vi "test5.vi"() -> ()   [LabVIEW 2014]
panel:
  out "In Range?":bool
  out "x-y":u32
  out "millisecond timer value 2":u32
  out "element":u32
  out "s? t:f 3":string
  out "s? t:f 2":string
  out "s? t:f":string
  out "appended array":u32[](array[numeric])
  out "millisecond timer value":u32
  in  "stop 2":bool
  out "String":string="3"
  out "Boolean 3":bool
  out "Boolean 2":bool
  out "Boolean":bool
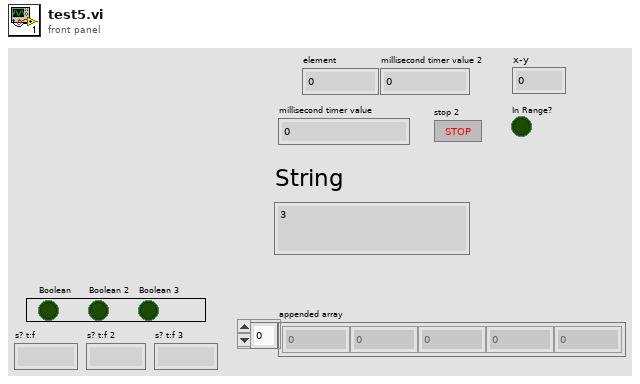
[diagram p1: front panel]
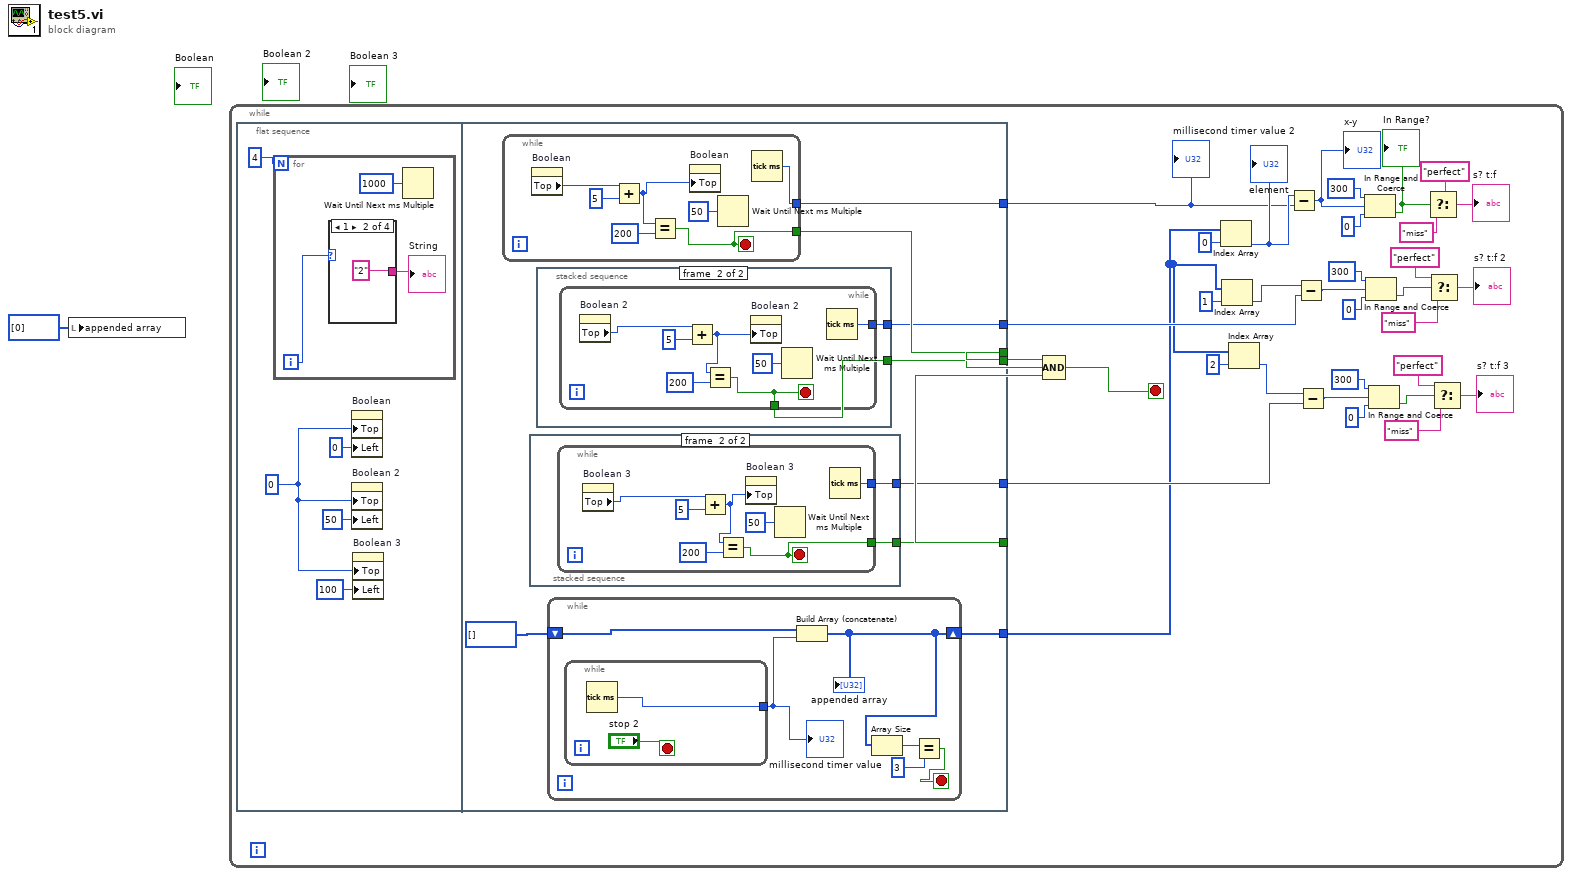
[diagram p0: block diagram]
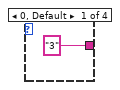
[diagram p2: hidden frame]
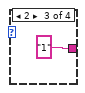
[diagram p3: hidden frame]
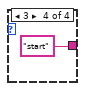
[diagram p4: hidden frame]
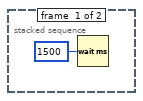
[diagram p5: hidden frame]
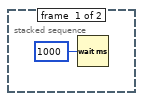
[diagram p6: hidden frame]
diagram:
  n1 = local write "appended array"(u32[] [0] ("appended array")) -> ()
  n2 = while {
    stop <- w33 stop-if-true
    n3 = flat-sequence {
      tunnel: [w56] -> w36
      tunnel: [w55] -> w35
      tunnel: [w54] -> w34
      tunnel: [w53] -> w28
      tunnel: [w52] -> w27
      tunnel: [w51] -> w25
      tunnel: [w49] -> w2
      frame #0 {
        w39 = 0
        n4 = for {
          N: 4 -> [_]
          i -> [w44]
          n5 = case shown="1" w44 {
            tunnel: ["3" "2" "1" "start"] -> w42
            frame 0, Default {
            }
            frame 1 {
            }
            frame 2 {
            }
            frame 3 {
            }
          }
          "String" <- w42
          n6 = Wait Until Next ms Multiple(millisecond multiple=u32 1000) -> ()  [unwired: 1 out]
        }
        n7 = property on="Boolean" class="Bool (strict)"("Top"=w39, "Left"=0 ("Position:Left")) -> ()  [unwired: 2 in, 2 out]
        n8 = property on="Boolean 2" class="Bool (strict)"("Top"=w39, "Left"=50 ("Position:Left")) -> ()  [unwired: 2 in, 2 out]
        n9 = property on="Boolean 3" class="Bool (strict)"("Top"=w39, "Left"=100 ("Position:Left")) -> ()  [unwired: 2 in, 2 out]
      }
      frame #1 {
        n10 = while {
          tunnel: [w86] -> w56
          tunnel: [w85] -> w53
          stop <- w86 stop-if-true
          n11 = property on="Boolean" class="Bool (strict)"() -> ("Top"=w90:i32)  [unwired: 2 in, 2 out]
          n12 = Add(x=w90, y=5) -> (x+y=w88:i32)
          n13 = Equal?(x=w88, y=200) -> (x = y?=w86:bool)
          n14 = property on="Boolean" class="Bool (strict)"("Top"=w88) -> ()  [unwired: 2 in, 2 out]
          n15 = Wait Until Next ms Multiple(millisecond multiple=u32 50) -> ()  [unwired: 1 out]
          n16 = Tick Count (ms)() -> (millisecond timer value=w85:u32)
        }
        n17 = stacked-sequence {
          tunnel: [_ w67] -> w54
          tunnel: [_ w66] -> w51
          frame #0 {
            n18 = Wait (ms)(milliseconds to wait=u32 1500) -> ()  [unwired: 1 out]
          }
          frame #1 {
            n19 = while {
              tunnel: [w70] -> w67
              tunnel: [w68] -> w66
              stop <- w70 stop-if-true
              n20 = property on="Boolean 3" class="Bool (strict)"() -> ("Top"=w71:i32)  [unwired: 2 in, 2 out]
              n21 = Add(x=w71, y=5) -> (x+y=w69:i32)
              n22 = Equal?(x=w69, y=200) -> (x = y?=w70:bool)
              n23 = property on="Boolean 3" class="Bool (strict)"("Top"=w69) -> ()  [unwired: 2 in, 2 out]
              n24 = Wait Until Next ms Multiple(millisecond multiple=u32 50) -> ()  [unwired: 1 out]
              n25 = Tick Count (ms)() -> (millisecond timer value=w68:u32)
            }
          }
        }
        n26 = stacked-sequence {
          tunnel: [_ w77] -> w55
          tunnel: [_ w76] -> w52
          frame #0 {
            n27 = Wait (ms)(milliseconds to wait=u32 1000) -> ()  [unwired: 1 out]
          }
          frame #1 {
            n28 = while {
              tunnel: [w79] -> w77
              tunnel: [w78] -> w76
              stop <- w79 stop-if-true
              n29 = property on="Boolean 2" class="Bool (strict)"() -> ("Top"=w82:i32)  [unwired: 2 in, 2 out]
              n30 = Add(x=w82, y=5) -> (x+y=w80:i32)
              n31 = Equal?(x=w80, y=200) -> (x = y?=w79:bool)
              n32 = property on="Boolean 2" class="Bool (strict)"("Top"=w80) -> ()  [unwired: 2 in, 2 out]
              n33 = Wait Until Next ms Multiple(millisecond multiple=u32 50) -> ()  [unwired: 1 out]
              n34 = Tick Count (ms)() -> (millisecond timer value=w78:u32)
            }
          }
        }
        n35 = while {
          shift-right: [w60] -> w49
          shift-left: u32[] [] -> [w62]
          stop <- w57 stop-if-true
          n36 = while {
            tunnel: [w63] -> w61
            stop <- "stop 2" stop-if-true
            n37 = Tick Count (ms)() -> (millisecond timer value=w63:u32)
          }
          "millisecond timer value" <- w61
          n38 = Build Array (concatenate)(w62, w61) -> (w60:u32[])
          "appended array" <- w60
          n39 = Array Size(array=w60) -> (size(s)=w59:i32)
          n40 = Equal?(x=w59, y=3) -> (x = y?=w57:bool)
        }
      }
    }
    n41 = Compound Arithmetic op=AND(w36, w35, w34) -> (w33:bool)
    n42 = Index Array(array=w2, index=0) -> (element=w29:u32)
    "element" <- w29
    n43 = Index Array(array=w2, index=1) -> (element=w26:u32)
    n44 = Index Array(array=w2, index=2) -> (element=w24:u32)
    n45 = Subtract(x=w29, y=w28) -> (x-y=w23:u32)
    "x-y" <- w23
    n46 = Subtract(x=w26, y=w27) -> (x-y=w4:u32)
    n47 = Subtract(x=w24, y=w25) -> (x-y=w3:u32)
    n48 = In Range and Coerce(upper limit=u32 300, x=w23, lower limit=u32 0) -> (In Range?=w20:bool)  [unwired: 1 out]
    "In Range?" <- w20
    n49 = In Range and Coerce(upper limit=u32 300, x=w4, lower limit=u32 0) -> (In Range?=w13:bool)  [unwired: 1 out]
    n50 = In Range and Coerce(upper limit=u32 300, x=w3, lower limit=u32 0) -> (In Range?=w8:bool)  [unwired: 1 out]
    n51 = Select(t="perfect", s=w20, f="miss") -> (s? t:f=→"s? t:f":string)
    n52 = Select(t="perfect", s=w13, f="miss") -> (s? t:f=→"s? t:f 2":string)
    n53 = Select(t="perfect", s=w8, f="miss") -> (s? t:f=→"s? t:f 3":string)
    "millisecond timer value 2" <- w28
  }
